vi "Measurement Query.vi"(0 "RedPitaya connection in":refnum<k5>, 2 "Query setting":u16(ring) items=["Vpp", "Mean voltage", "Max voltage", "Min voltage", "Signal frequency", "Signal period", "Duty cycle"], 5 "error in":errorcluster, 8 "Channel #":u16(ring) items=["Channel 1", "Channel 2"], 12 "timeout ms (2000)":i32) -> (14 "RedPitaya connection out":refnum<k5>, 16 "Output string":string, 19 "error out":errorcluster)   [LabVIEW 8.6]
doc: "Returns specific information about signal measurement from Red Pitaya."
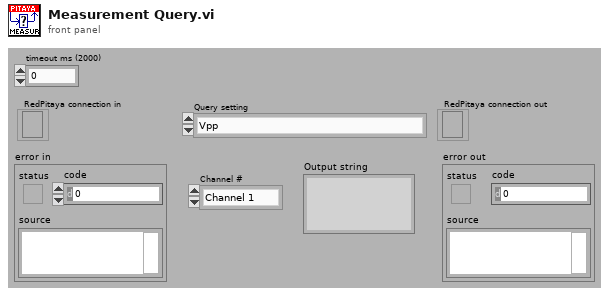
[diagram p1: front panel]
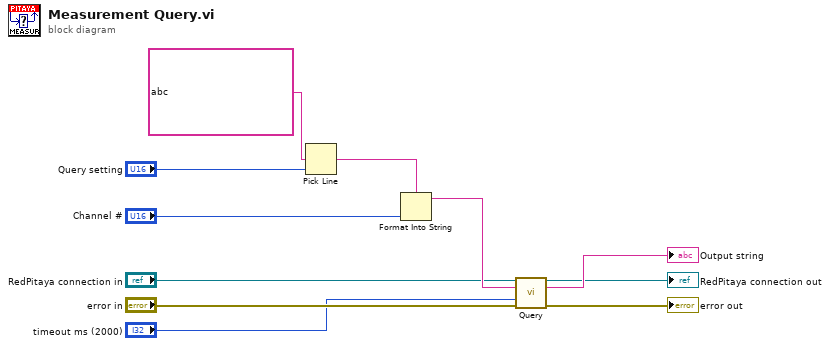
[diagram p0: block diagram]
diagram:
  n1 = Pick Line(multi-line string=string ?, line index="Query setting") -> (output string=w7:string)  [unwired: 1 in]
  n2 = Format Into String(format string=w7, "Channel #") -> (resulting string=w9:string)  [unwired: 2 in, 1 out]
  n3 = call "Query.vi"("RedPitaya connection in"="RedPitaya connection in", "SCPI Query"=w9, "timeout ms (2000)"="timeout ms (2000)", "error in"="error in") -> ("RedPitaya connection out"=→"RedPitaya connection out":refnum<k5>, "data out"=→"Output string":string, "error out"=→"error out":errorcluster)  [unwired: 9 in]
